vi "Read Step.vi"(8 "error in (no error)":errorcluster, 11 "IV_meas in":refnum<class "IV_meas.lvclass">) -> (0 "error out":errorcluster, 2 "Step":dbl, 3 "IV_meas out":refnum<class "IV_meas.lvclass">)   [LabVIEW 2014, in "IV_meas.lvclass"]
uses:
  IV_meas.lvclass
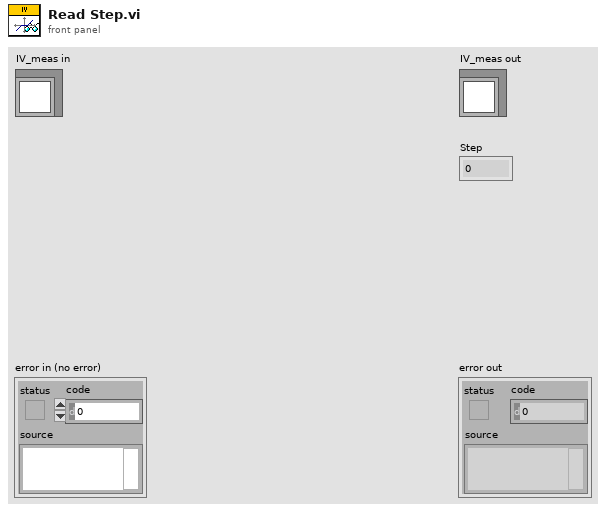
[diagram p1: front panel]
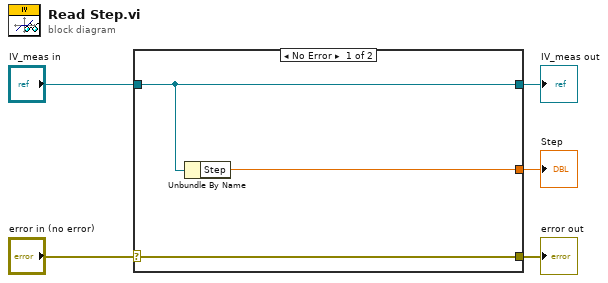
[diagram p0: block diagram]
diagram:
  n1 = case shown="No Error" "error in (no error)" {
    selector: "error in (no error)" -> [w8 w9]
    tunnel: [w8 w9] -> w4
    tunnel: [w7 w10] -> w2
    tunnel: "IV_meas in" -> [w7 w10]
    tunnel: [w6 _] -> w1
    frame No Error {
      n2 = Unbundle By Name(w7) -> ("Step"=w6:dbl)
    }
    frame Error {
    }
  }
  "error out" <- w4
  "IV_meas out" <- w2
  "Step" <- w1
